vi "Add section.vi"(8 "error in":errorcluster, 10 "Label.Text in":string, 11 "Data in":T2 {"Device Ref" format="%.0x"; "Section Ref" format="%.0x"}) -> (0 "error out":errorcluster, 1 "Section Ptr":T1=18446744073709551615 format="%.0x", 2 "Item Name":string, 3 "Data out":T2 {"Device Ref" format="%.0x"; "Section Ref" format="%.0x"})   [LabVIEW 2016, in "DCM System Explorer.lvlib"]
uses:
  DCM System Explorer.lvlib
  <vilib>/NI Veristand/Custom Device API/Custom Device Item Ref.ctl
  <vilib>/NI VeriStand/Custom Device API/Custom Device API.lvlib
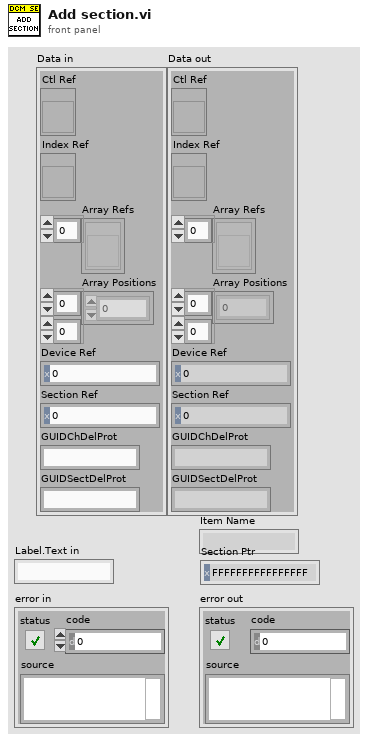
[diagram p1: front panel]
types:
  T1 = typedef "Custom Device API.lvlib/Custom Device Item Ref.ctl" = u64
  T2 = cluster{"Ctl Ref":refnum<vi>, "Index Ref":refnum<vi>, "Array Refs":refnum<vi>[], "Array Positions":i32[][], "Device Ref":T1, "Section Ref":T1, "GUIDChDelProt":string, "GUIDSectDelProt":string}
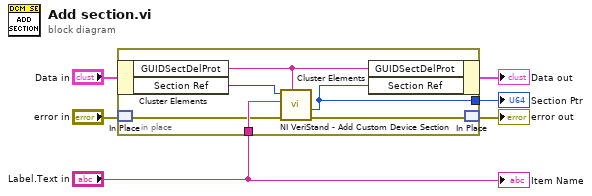
[diagram p0: block diagram]
diagram:
  n1 = in-place {
    in-place-border: "Label.Text in" -> [w10]
    in-place-border: [w7] -> w1
    n2 = in-place-cluster #1("Data in") -> ("GUIDSectDelProt"=w11:string, "Section Ref"=w12:T1)
    n3 = in-place-match #2("error in") -> (w9:errorcluster)
    n4 = call <vilib>:"NI VeriStand - Add Custom Device Section.vi"("GUID (Default Section)"=w11, "error in (no error)"=w9, "Section Name"=w10, "Parent Ref in"=w12) -> ("error out"=w8:errorcluster, "Section Ptr"=w7:T1)  [unwired: 4 in, 2 out]
    n5 = in-place-cluster #1("GUIDSectDelProt"=w11, "Section Ref"=w7) -> (→"Data out":T2)
    n6 = in-place-match #2(w8) -> (→"error out":errorcluster)
  }
  "Section Ptr" <- w1
  "Item Name" <- "Label.Text in"
